vi "scale.vi"(11 "Yaw":dbl) -> (3 "Scaled Yaw":dbl)   [LabVIEW 2015, in "Nav6.lvlib"]
uses:
  Nav6.lvlib
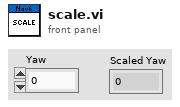
[diagram p1: front panel]
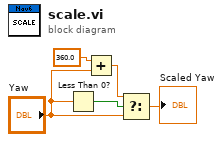
[diagram p0: block diagram]
diagram:
  n1 = Less Than 0?(x="Yaw") -> (x < 0?=w5:bool)
  n2 = Add(x=360.0, y="Yaw") -> (x+y=w4:dbl)
  n3 = Select(t=w4, s=w5, f="Yaw") -> (s? t:f=→"Scaled Yaw":dbl)
